vi "LSX Get Hand Wheel.vi"(7 "pbEncoder":i32, 8 "error in (no error)":errorcluster, 9 "pbPositionCount":i32, 10 "pbHandWheelOn":i32, 11 "lLSID":i32) -> (0 "error out":errorcluster, 1 "pbPositionCount out":i32, 2 "pbHandWheelOn out":i32, 3 "function return":i32, 5 "pbEncoder out":i32)   [LabVIEW 2016, in "Tango_DLL.lvlib"]
doc: "TANGOAPI int TANGOCALL LSX_GetHandWheel (int lLSID, BOOL *pbHandWheelOn, BOOL *pbPositionCount, BOOL *pbEncoder);"
uses:
  Tango_DLL.lvlib
  2017/Microscope Control/Device Library/Stages/Marzhauser/SCAN IM 120 x 80/Tango DLL VIs/Tango_DLL.dll
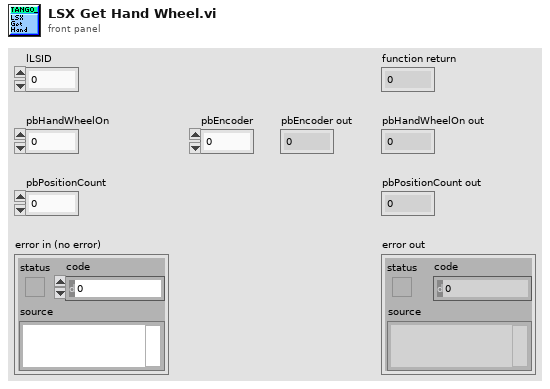
[diagram p1: front panel]
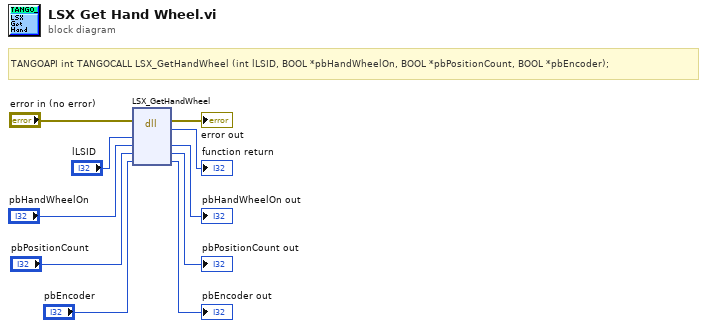
[diagram p0: block diagram]
diagram:
  # "TANGOAPI int TANGOCALL LSX_GetHandWheel (int lLSID, BOOL *pbHandWheelOn, BOOL *pbPositionCount, BOOL *pbEncoder);"
  n1 = dll-call lib="C:/Users/4PiSMS/Documents/Microscope Control/2017/Microscope Control/Device Library/Stages/Marzhauser/SCAN IM 120 x 80/Tango DLL VIs/Tango_DLL.*" fn="LSX_GetHandWheel"(error in="error in (no error)", "lLSID"="lLSID", "pbHandWheelOn"="pbHandWheelOn", "pbPositionCount"="pbPositionCount", "pbEncoder"="pbEncoder") -> (error out=→"error out":errorcluster, →"function return":i32, "pbHandWheelOn"=→"pbHandWheelOn out":i32, "pbPositionCount"=→"pbPositionCount out":i32, "pbEncoder"=→"pbEncoder out":i32)  [unwired: 3 in, 1 out]
